vi "TCP_load_test.vi"() -> ()   [LabVIEW 2010]
uses:
  <vilib>/ptbypt/NI_PtbyPt.lvlib
panel:
  in  "Path":path=path "Z:/Experiments/spinorbec/imaging test/20120120T143000_trigger_camera_on_imaging_beam_0.h5"
  out "stddev":dbl format="%0.2f"
  out "mean":dbl format="%0.2f"
  out "Waveform Chart":u32(graph)
  in  "stop":bool
  out "exec time":u32
  out "error out":errorcluster
  out "state":string
  out "resp2":string
  out "resp1":string
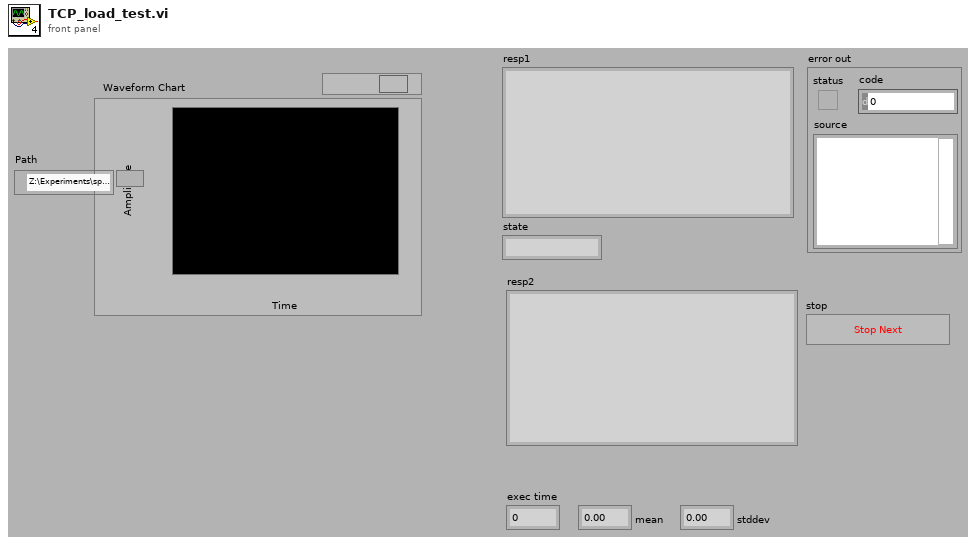
[diagram p1: front panel]
types:
  T1 = enum16{"Standard", "Buffered", "CRLF", "Immediate"}
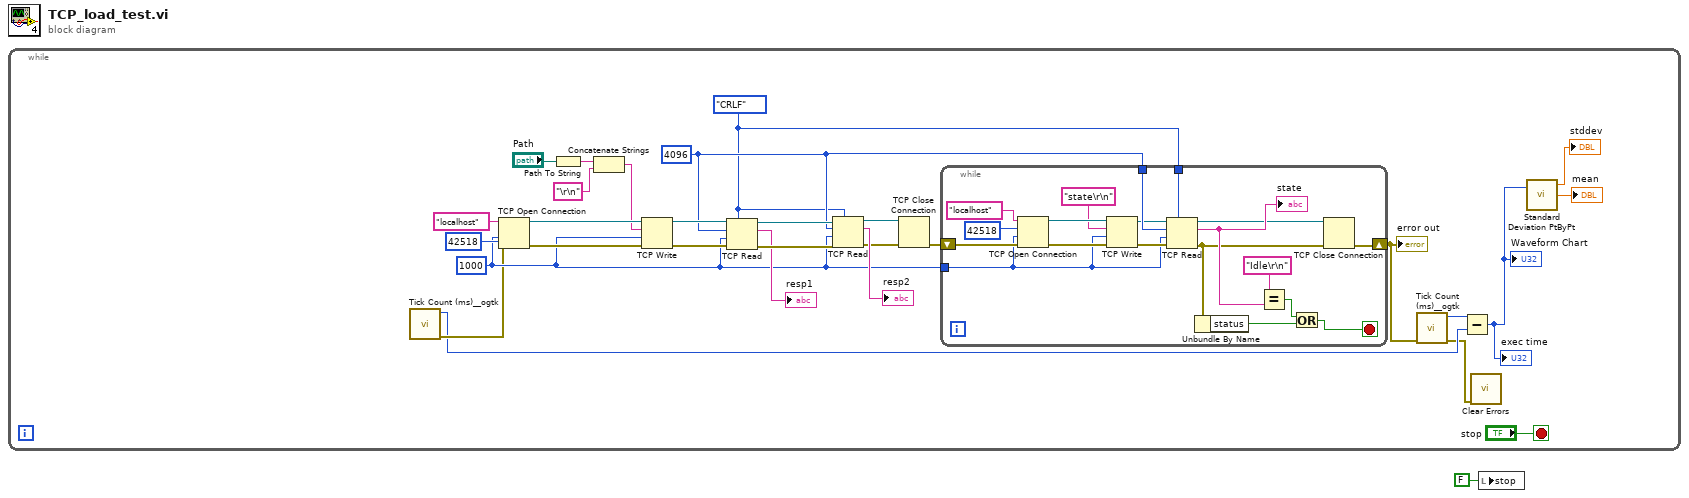
[diagram p0: block diagram]
diagram:
  n1 = while {
    stop <- "stop" stop-if-true
    w16 = 4096 ("bytes to read")
    w15 = T1."CRLF" ("mode (standard)")
    w17 = 1000 ("timeout ms (25000)")
    n2 = call <userlib>:"Tick Count (ms)__ogtk.vi"() -> ("error out"=w14:errorcluster, "millisecond timer value"=w11:u32)  [unwired: 10 in]
    n3 = TCP Open Connection(address="localhost", remote port or service name=u16 42518, timeout ms (60000)=w17, error in (no error)=w14) -> (connection ID=w28:refnum<k5>, error out=w27:errorcluster)  [unwired: 1 in]
    n4 = Path To String(path="Path") -> (string=w4:string)
    n5 = Concatenate Strings(w4, "\r\n" ("data in")) -> (w2:string)
    n6 = TCP Write(connection ID=w28, data in=w2, error in (no error)=w27, 9:w17) -> (connection ID out=w26:refnum<k5>, error out=w25:errorcluster)  [unwired: 1 out]
    n7 = TCP Read(connection ID=w26, bytes to read=w16, error in (no error)=w25, 7:w15, 9:w17) -> (connection ID out=w24:refnum<k5>, data out=→"resp1":string, error out=w23:errorcluster)
    n8 = TCP Read(connection ID=w24, bytes to read=w16, error in (no error)=w23, 7:w15, 9:w17) -> (connection ID out=w20:refnum<k5>, data out=→"resp2":string, error out=w19:errorcluster)
    n9 = TCP Close Connection(connection ID=w20, error in (no error)=w19) -> (error out=w18:errorcluster)  [unwired: 1 in, 1 out]
    n10 = while {
      tunnel: w17 -> [w31]
      tunnel: w16 -> [w44]
      tunnel: w15 -> [w43]
      shift-right: [w33] -> w13
      shift-left: w18 -> [w47]
      stop <- w32 stop-if-true
      n11 = TCP Open Connection(address="localhost", remote port or service name=u16 42518, timeout ms (60000)=w31, error in (no error)=w47) -> (connection ID=w46:refnum<k5>, error out=w45:errorcluster)  [unwired: 1 in]
      n12 = TCP Write(connection ID=w46, data in="state\r\n", error in (no error)=w45, 9:w31) -> (connection ID out=w41:refnum<k5>, error out=w40:errorcluster)  [unwired: 1 out]
      n13 = TCP Read(connection ID=w41, bytes to read=w44, error in (no error)=w40, 7:w43, 9:w31) -> (connection ID out=w35:refnum<k5>, data out=w37:string, error out=w34:errorcluster)
      "state" <- w37
      n14 = Unbundle By Name(w34) -> ("status"=w39:bool)
      n15 = Equal?(x="Idle\r\n" ("data out"), y=w37) -> (x = y?=w36:bool)
      n16 = Or(x=w36, y=w39) -> (x .or. y?=w32:bool)
      n17 = TCP Close Connection(connection ID=w35, error in (no error)=w34) -> (error out=w33:errorcluster)  [unwired: 1 in, 1 out]
    }
    "error out" <- w13
    n18 = call <userlib>:"Tick Count (ms)__ogtk.vi"("error in (no error)"=w13) -> ("error out"=w6:errorcluster, "millisecond timer value"=w12:u32)  [unwired: 9 in]
    n19 = Subtract(x=w12, y=w11) -> (x-y=w9:u32)
    "exec time" <- w9
    "Waveform Chart" <- w9
    n20 = call <vilib>:"Clear Errors.vi"("error in (no error)"=w6) -> ()  [unwired: 6 in, 1 out]
    n21 = call <vilib>:"Standard Deviation PtByPt.vi"("x"=w9) -> ("standard deviation"=→"stddev":dbl, "mean"=→"mean":dbl)  [unwired: 2 in, 1 out]
  }
  n22 = local write "stop"(FALSE ("stop")) -> ()
